vi "Subvi DO detector.vi"(2 "DO":refnum<k21>="Connector0/DIO5", 10 "Memory label":refnum<k21>="Gate buffer") -> ()   [LabVIEW 2017]
uses:
  <vilib>/rvi/DataTransferAndStorage/Container/Common/niFpgaContainerExecOnDevCompGetState.vi
  <vilib>/rvi/Emulation/niFpgaEmulationIsFPGAContextNoSignature.vi
  <vilib>/rvi/DataTransferAndStorage/Container/Common/niFpgaContainerGetUniqueNameForEmu.vi
  <vilib>/rvi/Emulation/niFpgaProcessEmulError.vi
  <vilib>/rvi/Emulation/niFpgaSctlEmulationGetInTimedLoop.vi
  <vilib>/rvi/errors/nirviReportUnexpectedCaseInternalError (U32).vi
  <vilib>/rvi/Memory/Memory_Emulation/niFpgaMemoryEmulationCacheClearOnFirstRun.vi
  <vilib>/rvi/Memory/Memory_Emulation/nirvimemoryEmulationManagerCache_MakeExclusive.vi
  <vilib>/rvi/Memory/Memory_Emulation/niFpgaMemoryEmulationValidateCache.vi
  <vilib>/rvi/Memory/Memory_Emulation/nirvimemoryEmulationManagerCache_InsertValue.vi
  <vilib>/Utility/error.llb/Clear Errors.vi
  <vilib>/rvi/Memory/Memory_Emulation/nirvimemoryEmulationManagerCache_ReleaseExclusive.vi
  <vilib>/rvi/Memory/Memory_Emulation/nirvimemoryEmulationManagerCache_GetValue.vi
  <vilib>/rvi/Memory/Memory_Emulation/nirvimemoryEmulationManagerCache_SetValue.vi
  <vilib>/rvi/Emulation/niFpgaSctlEmulationResourceMgr.vi
  GV gating.vi
  <vilib>/rvi/eio/common/nirviEmuTemplateMethod_errors.vi
  <vilib>/rvi/DataTransferAndStorage/Container/XNode/niFpgaContainer.xnode
  <vilib>/rvi/Memory/Memory_Emulation/niFpgaMemoryEmulationRefIn.vi
  <vilib>/eio/EIONode/EIONode.xnode
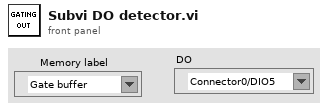
[diagram p1: front panel]
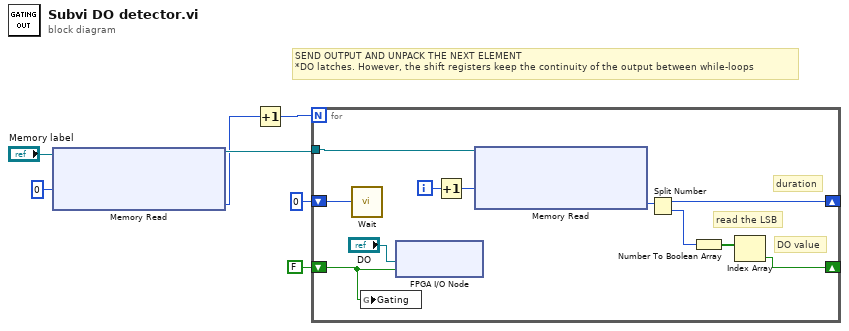
[diagram p0: block diagram]
diagram:
  # "SEND OUTPUT AND UNPACK THE NEXT ELEMENT\n*DO latches. However, the shift registers keep the continuity of the output between while-loops"
  n1 = xnode ("Memory Read")("Address"=u32 0, "Memory In"="Memory label") -> ("Data"=w5:u32, "Memory Out"=w7:refnum<k21>)
  n2 = Increment(x=w5) -> (x+1=w6:u32)
  n3 = for {
    N: w6 -> [_]
    shift-right: [w13] -> _
    shift-left: FALSE -> [w8]
    shift-right: [w15] -> _
    shift-left: u16 0 -> [w14]
    tunnel: w7 -> [w10]
    i -> [w12]
    # "read the LSB"
    # "DO value"
    # "duration"
    n4 = call "Wait"("Count(Ticks)"=w14) -> ()  [unwired: 1 out]
    n5 = global write "GV gating.vi" "Gating"(w8) -> ()
    n6 = xnode "FPGA I/O Node"("I/O Item"=w8, "FPGA I/O In"="DO") -> ()  [unwired: 1 out]
    n7 = Increment(x=w12) -> (x+1=w11:i32)
    n8 = xnode ("Memory Read")("Address"=w11, "Memory In"=w10) -> ("Data"=w17:u32)  [unwired: 1 out]
    n9 = Split Number(x=w17) -> (hi(x)=w15:u16, lo(x)=w16:u16)
    n10 = Number To Boolean Array(number=w16) -> (Boolean array=w18:bool[])
    n11 = Index Array(array=w18) -> (element=w13:bool)  [unwired: 1 in]
  }
